vi "Calculate dx of Uneven X.vi"(10 "Y In":dbl[](array[numeric]), 11 "X":dbl[](array[numeric])) -> (0 "error":i32, 2 "Y out":dbl[](array[numeric]), 3 "delta X":dbl[](array[numeric]))   [LabVIEW 2020, in "NI_AALPro.lvlib"]
uses:
  NI_AALPro.lvlib
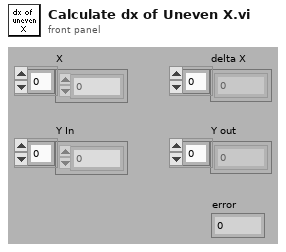
[diagram p1: front panel]
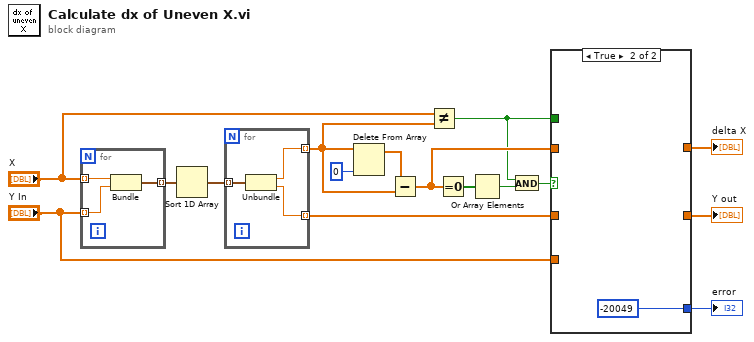
[diagram p0: block diagram]
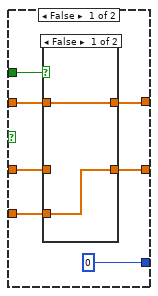
[diagram p2: hidden frame]
diagram:
  n1 = for {
    tunnel: "Y In" -> [w18] mode=indexing
    tunnel: "X" -> [w19] mode=indexing
    tunnel: [w17] -> w16 mode=indexing
    n2 = Bundle("Numeric"=w19, "Numeric"=w18) -> (w17:cluster{"Numeric":dbl, "Numeric":dbl})  [unwired: 1 in]
  }
  n3 = Sort 1D Array(array=w16) -> (sorted array=w15:cluster{"Numeric":dbl, "Numeric":dbl}[])
  n4 = for {
    tunnel: w15 -> [w22] mode=indexing
    tunnel: [w21] -> w4 mode=indexing
    tunnel: [w20] -> w9 mode=indexing
    n5 = Unbundle(w22) -> ("Numeric"=w21:dbl, "Numeric"=w20:dbl)
  }
  n6 = Delete From Array(array=w4, index=0) -> (array with subset deleted=w2:dbl[])  [unwired: 1 in, 1 out]
  n7 = Subtract(x=w2, y=w4) -> (x-y=w5:dbl[])
  n8 = Not Equal?(x="X", y=w4) -> (x != y?=w1:bool)
  n9 = Equal To 0?(x=w5) -> (x = 0?=w14:bool[])
  n10 = Or Array Elements(Boolean array=w14) -> (logical OR=w12:bool)
  n11 = And(x=w1, y=w12) -> (x .and. y?=w11:bool)
  n12 = case shown="True" w11 {
    tunnel: w1 -> [w29 _]
    tunnel: w5 -> [w28 _]
    tunnel: "Y In" -> [w27 _]
    tunnel: w9 -> [w26 _]
    tunnel: [w25 _] -> w8
    tunnel: [w24 _] -> w7
    tunnel: [0 -20049] -> w6
    frame False {
      n13 = case shown="False" w29 {
        tunnel: w28 -> [w30 w33]
        tunnel: w27 -> [w31 _]
        tunnel: [w31 w32] -> w24
        tunnel: [w30 w33] -> w25
        tunnel: w26 -> [_ w32]
        frame False {
        }
        frame True {
        }
      }
    }
    frame True {
    }
  }
  "delta X" <- w8
  "Y out" <- w7
  "error" <- w6
